vi "Read Behaviour Tree.vi"(8 "error in (no error)":errorcluster, 11 "bt_System in":refnum<class "bt_System.lvclass">) -> (0 "error out":errorcluster, 2 "BT.lvlib:bt_Node.lvclass":refnum<class "bt_Node.lvclass">, 3 "bt_System out":refnum<class "bt_System.lvclass">)   [LabVIEW 2021, in "BT.lvlib" / "bt_System.lvclass"]
uses:
  bt_System.lvclass
  bt_System.lvclass/bt_System.ctl
  Support/Nodes/abs_Node/bt_Node.lvclass
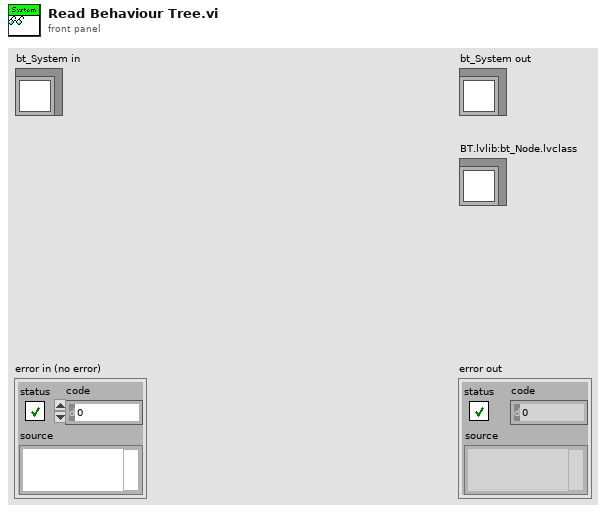
[diagram p1: front panel]
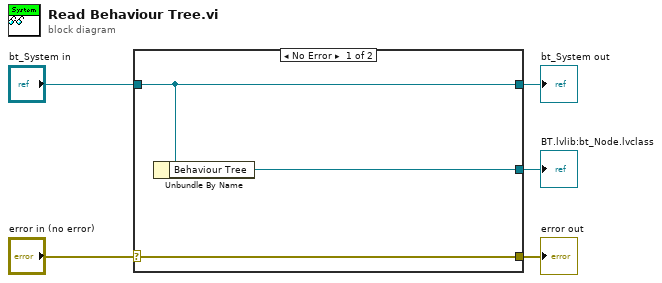
[diagram p0: block diagram]
diagram:
  n1 = case shown="No Error" "error in (no error)" {
    selector: "error in (no error)" -> [w8 w9]
    tunnel: [w8 w9] -> w4
    tunnel: [w7 w10] -> w2
    tunnel: "bt_System in" -> [w7 w10]
    tunnel: [w6 _] -> w1
    frame No Error {
      n2 = Unbundle By Name(w7) -> ("Behaviour Tree"=w6:refnum<class "bt_Node.lvclass">)
    }
    frame Error {
    }
  }
  "error out" <- w4
  "bt_System out" <- w2
  "BT.lvlib:bt_Node.lvclass" <- w1
